vi "3过0插值法子程序.vi"(1 "波形":waveform(dbl)) -> (0 "f":dbl)   [LabVIEW 2017]
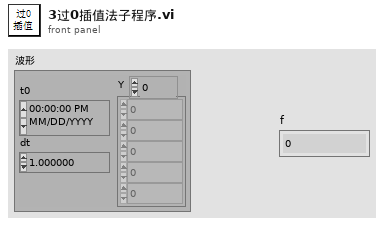
[diagram p1: front panel]
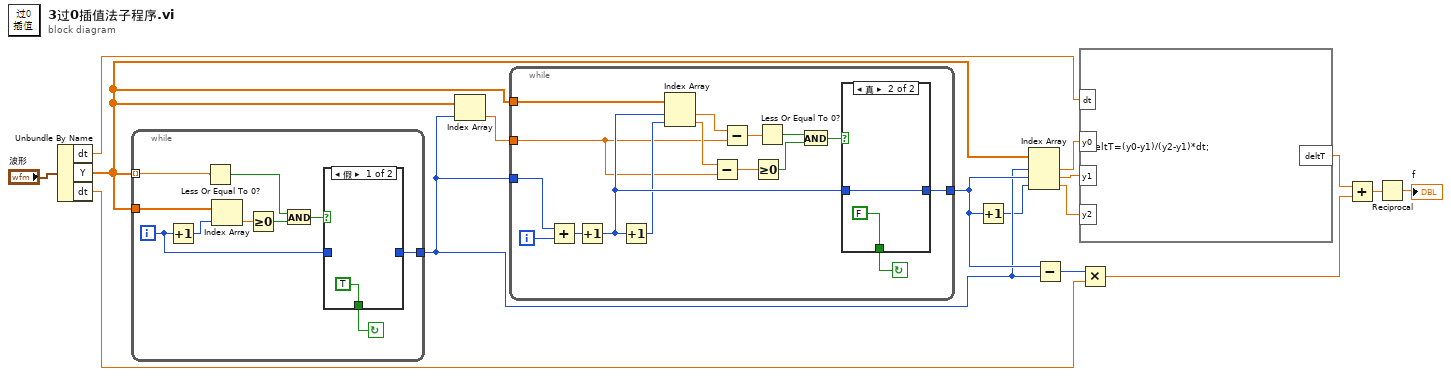
[diagram p0: block diagram]
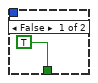
[diagram p2: hidden frame]
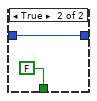
[diagram p3: hidden frame]
diagram:
  n1 = Unbundle By Name("波形") -> ("dt"=w9:dbl, "Y"=w3:dbl[], "dt"=w6:dbl)
  n2 = while {
    tunnel: w3 -> [w23] mode=indexing
    tunnel: w3 -> [w26]
    tunnel: [w18] -> w8
    i -> [w19]
    stop <- w17 continue-if-true
    n3 = Increment(x=w19) -> (x+1=w25:i32)
    n4 = Less Or Equal To 0?(x=w23) -> (x <= 0?=w21:bool)
    n5 = Index Array(array=w26, index=w25) -> (element=w24:dbl)
    n6 = Greater Or Equal To 0?(x=w24) -> (x >= 0?=w22:bool)
    n7 = And(x=w21, y=w22) -> (x .and. y?=w20:bool)
    n8 = case shown="假" w20 {
      tunnel: w19 -> [_ w29]
      tunnel: [_ w29] -> w18
      tunnel: [TRUE FALSE] -> w17
      frame False {
      }
      frame True {
      }
    }
  }
  n9 = Index Array(array=w3, index=w8) -> (element=w10:dbl)
  n10 = while {
    tunnel: w3 -> [w45]
    tunnel: [w39] -> w15
    tunnel: w8 -> [w37]
    tunnel: w10 -> [w30]
    i -> [w36]
    stop <- w38 continue-if-true
    n11 = Add(x=w37, y=w36) -> (x+y=w35:i32)
    n12 = Increment(x=w35) -> (x+1=w34:i32)
    n13 = Increment(x=w34) -> (x+1=w33:i32)
    n14 = Index Array(array=w45, index #1=w34, index #2=w33) -> (element #1=w32:dbl, element #2=w31:dbl)
    n15 = Subtract(x=w31, y=w30) -> (x-y=w43:dbl)
    n16 = Subtract(x=w32, y=w30) -> (x-y=w44:dbl)
    n17 = Greater Or Equal To 0?(x=w43) -> (x >= 0?=w41:bool)
    n18 = Less Or Equal To 0?(x=w44) -> (x <= 0?=w42:bool)
    n19 = And(x=w42, y=w41) -> (x .and. y?=w40:bool)
    n20 = case shown="真" w40 {
      tunnel: w34 -> [_ w48]
      tunnel: [_ w48] -> w39
      tunnel: [TRUE FALSE] -> w38
      frame False {
      }
      frame True {
      }
    }
  }
  n21 = Increment(x=w15) -> (x+1=w5:i32)
  n22 = Index Array(array=w3, index #1=w8, index #2=w15, index #3=w5) -> (element #1=w14:dbl, element #2=w2:dbl, element #3=w13:dbl)
  n23 = Subtract(x=w15, y=w8) -> (x-y=w7:i32)
  n24 = formula code="deltT=(y0-y1)/(y2-y1)*dt;"("y0"=w14, "y1"=w2, "y2"=w13, "dt"=w9) -> ("deltT"=w12:dbl)
  n25 = Multiply(x=w7, y=w6) -> (x*y=w1:dbl)
  n26 = Add(x=w12, y=w1) -> (x+y=w11:dbl)
  n27 = Reciprocal(x=w11) -> (1/x=→"f":dbl)
